vi "Read ZI Handle.vi"(8 "error in (no error)":errorcluster, 11 "ZI Lockin in":refnum<class "ZI Lockin.lvclass">) -> (0 "error out":errorcluster, 2 "ziHandle":T1 {"Handle" format="0x%08x"; "Conn" format="0x%08x"}, 3 "ZI Lockin out":refnum<class "ZI Lockin.lvclass">)   [LabVIEW 2016, in "ZI Lockin.lvclass"]
uses:
  ZI Lockin.lvclass
  Program Files/National Instruments/LabVIEW 2016/instr.lib/Zurich Instruments LabOne/Public/ziTypeHandle.ctl
  ZI Lockin.lvclass/ZI Lockin.ctl
  Program Files/National Instruments/LabVIEW 2016/instr.lib/Zurich Instruments LabOne/Zurich Instruments LabOne.lvlib
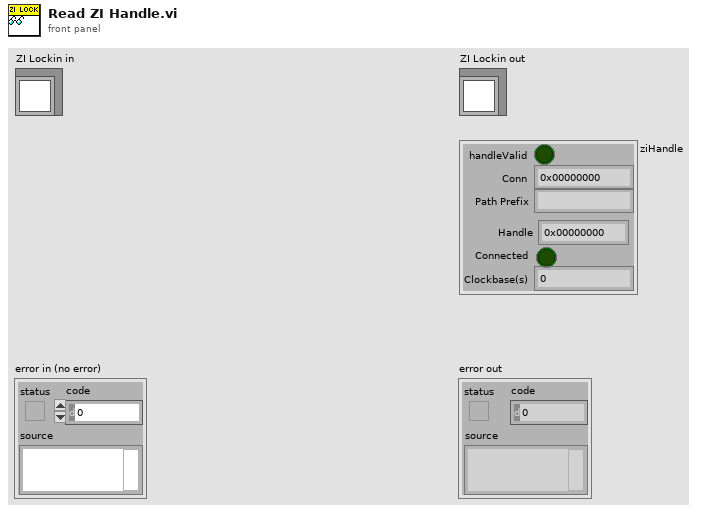
[diagram p1: front panel]
types:
  T1 = typedef "Zurich Instruments LabOne.lvlib/ziTypeHandle.ctl" = cluster{"handleValid":bool, "Conn":u64, "Path Prefix":string, "Handle":u64, "Connected":bool, "Clockbase(s)":dbl}
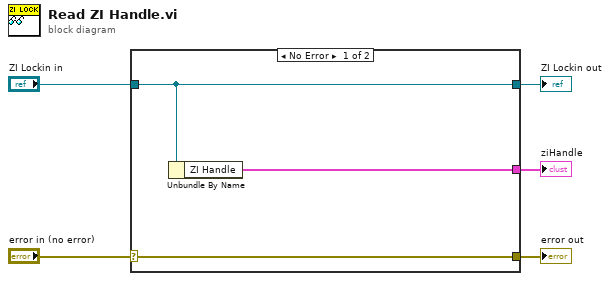
[diagram p0: block diagram]
diagram:
  n1 = case shown="No Error" "error in (no error)" {
    selector: "error in (no error)" -> [w8 w9]
    tunnel: [w8 w9] -> w4
    tunnel: [w7 w10] -> w2
    tunnel: "ZI Lockin in" -> [w7 w10]
    tunnel: [w6 _] -> w1
    frame No Error {
      n2 = Unbundle By Name(w7) -> ("ZI Handle"=w6:T1)
    }
    frame Error {
    }
  }
  "error out" <- w4
  "ZI Lockin out" <- w2
  "ziHandle" <- w1
